vi "ATSh_AbortAsyncRead.vi"(11 "Handle":u32) -> (0 "Return Code":u32)   [LabVIEW 2014]
doc: "_____AlazarTech, Scope_____\n\nAborts any in-progress transfers, and cancels any pending transfers on the board."
uses:
  ATSApi.dll
panel:
  out "Handle_Out":u32
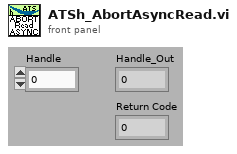
[diagram p1: front panel]
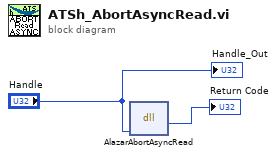
[diagram p0: block diagram]
diagram:
  n1 = dll-call lib="D:/IntensityOCT/trunk/ATSApi.dll" fn="AlazarAbortAsyncRead"("Handle"="Handle") -> (→"Return Code":u32)  [unwired: 4 in, 2 out]
  "Handle_Out" <- "Handle"
